vi "Scan.vi"(4 "with tracking (true)":bool=TRUE, 6 "attenuation, dB (0)":dbl, 7 "step, Hz":u32 format="%.0p", 8 "error in (no error)":errorcluster, 9 "end, Hz":u32 format="%.0p", 10 "start, Hz":u32 format="%.0p", 11 "Arinst SSA-TG in":refnum<class "PL Arinst SSA-TG.lvclass">) -> (0 "error out":errorcluster, 1 "scan time, ms":u32, 2 "scan data":T1, 3 "Arinst SSA-TG out":refnum<class "PL Arinst SSA-TG.lvclass">)   [LabVIEW 2015, in "PL Arinst SSA-TG.lvclass"]
doc: "Initiates frequency range scan and returns scan data and scan time."
uses:
  PL Arinst SSA-TG.lvclass
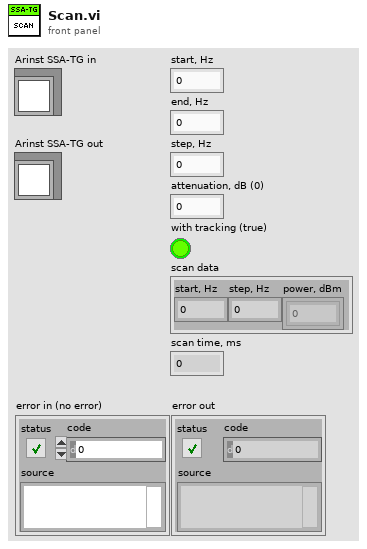
[diagram p1: front panel]
types:
  T1 = cluster{"start, Hz":u32, "step, Hz":u32, "power, dBm":dbl[]}
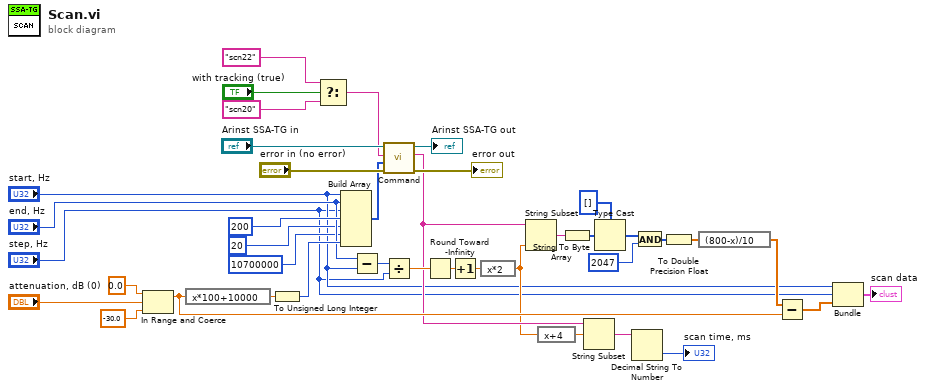
[diagram p0: block diagram]
diagram:
  n1 = In Range and Coerce(upper limit=0.0, x="attenuation, dB (0)", lower limit=-30.0) -> (coerced(x)=w10:dbl)  [unwired: 1 out]
  n2 = expression code="x*100+10000"(w10) -> (w33:dbl)
  n3 = To Unsigned Long Integer(number=w33) -> (unsigned 32bit integer=w31:u32)
  n4 = Select(t="scn22" ("command"), s="with tracking (true)", f="scn20" ("command")) -> (s? t:f=w27:string)
  n5 = Build Array("start, Hz", "end, Hz", "step, Hz", u32 200 ("element"), u32 20 ("element"), u32 10700000 ("element"), w31) -> (w26:u32[])
  n6 = Subtract(x="end, Hz", y="start, Hz") -> (x-y=w25:u32)
  n7 = call "Command.vi"("error in (no error)"="error in (no error)", "arguments (none)"=w26, "command"=w27, "Arinst SSA-TG in"="Arinst SSA-TG in") -> ("error out"=→"error out":errorcluster, "response data"=w7:string, "Arinst SSA-TG out"=→"Arinst SSA-TG out":refnum<class "PL Arinst SSA-TG.lvclass">)  [unwired: 5 in]
  n8 = Divide(x=w25, y="step, Hz") -> (x/y=w24:dbl)
  n9 = Round Toward -Infinity(1:w24) -> (0:w23:dbl)
  n10 = Increment(x=w23) -> (x+1=w21:dbl)
  n11 = expression code="x*2"(w21) -> (w6:dbl)
  n12 = String Subset(string=w7, length (rest)=w6) -> (substring=w12:string)  [unwired: 1 in]
  n13 = expression code="x+4"(w6) -> (w9:dbl)
  n14 = String To Byte Array(string=w12) -> (unsigned byte array=w17:u8[])
  n15 = String Subset(string=w7, offset (0)=w9) -> (substring=w8:string)  [unwired: 1 in]
  n16 = Type Cast(type=u16[] [] ("unsigned byte array"), x=w17) -> (*(type *) &x=w16:u16[])
  n17 = Decimal String To Number(string=w8) -> (number=→"scan time, ms":i32)  [unwired: 2 in, 1 out]
  n18 = And(x=w16, y=u16 2047) -> (x .and. y?=w14:u16[])
  n19 = To Double Precision Float(number=w14) -> (double precision float=w13:dbl[])
  n20 = expression code="(800-x)/10"(w13) -> (w11:dbl[])
  n21 = Subtract(x=w11, y=w10) -> (x-y=w4:dbl[])
  n22 = Bundle("start, Hz"="start, Hz", "step, Hz"="step, Hz", w4) -> (→"scan data":cluster{"start, Hz":u32, "step, Hz":u32, dbl[]})  [unwired: 1 in]
